vi "VS-Compute Heart Rate.vi"(0 "ECG":dbl[](array[numeric]), 7 "Sampling Rate (Hz)":dbl=10000.0, 11 "error in (no error)":errorcluster) -> (6 "Heart Rate (bpm)":dbl format="%.1f", 10 "XY Graph":cluster{"Array":dbl[], "Filtered X":dbl[]}[](graph), 15 "error out":errorcluster)   [LabVIEW 2020]
uses:
  <vilib>/Analysis/3filter.llb/Filter Passband Type.ctl
  epl-vi-lib/Utility VIs/Math VIs/LinSpace (x0-dx-npts).vi
  <vilib>/Analysis/baseanly.llb/Mean (DBL).vi
  <vilib>/Analysis/3filter.llb/Butterworth Filter (DBL).vi
  <vilib>/Analysis/NI_AALPro.lvlib
  <vilib>/Analysis/NI_AALBase.lvlib
  <vilib>/Analysis/NI_AAL_SigProc.lvlib
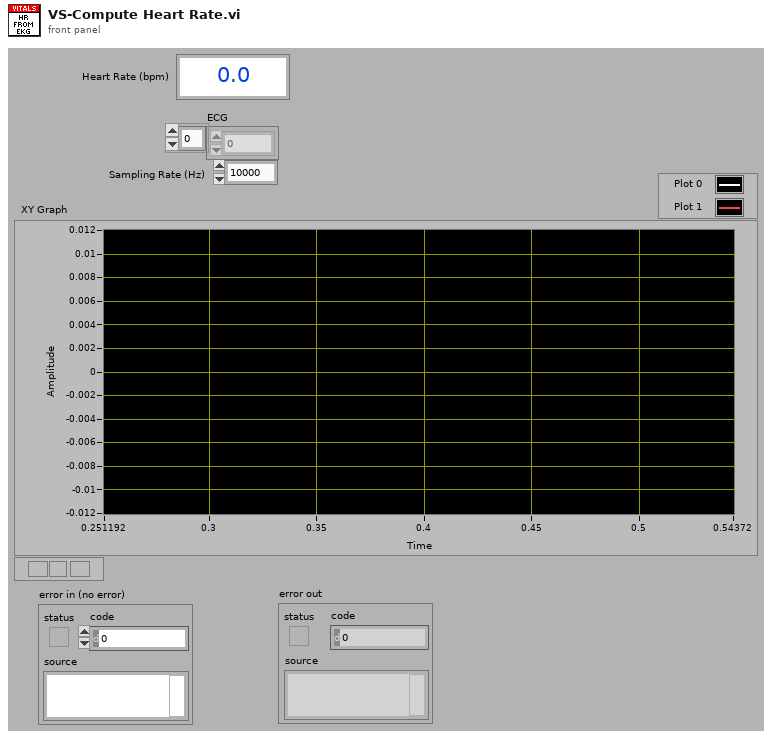
[diagram p1: front panel]
types:
  T1 = typedef "NI_AALBase.lvlib/Filter Passband Type.ctl" = enum32{"Lowpass", "Highpass", "Bandpass", "Bandstop"}
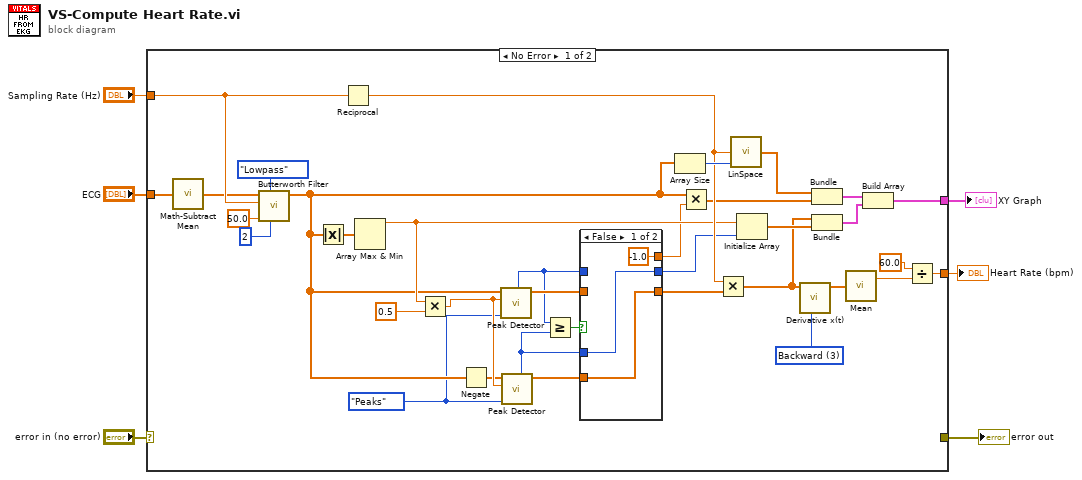
[diagram p0: block diagram]
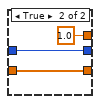
[diagram p2: hidden frame]
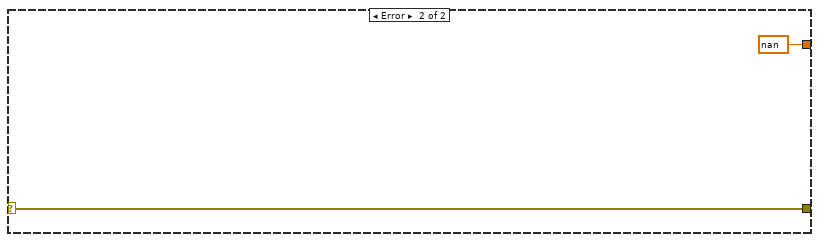
[diagram p3: hidden frame]
diagram:
  n1 = case shown="No Error" "error in (no error)" {
    selector: "error in (no error)" -> [_ w49]
    tunnel: [w41 nan] -> w6
    tunnel: "ECG" -> [w39 _]
    tunnel: "Sampling Rate (Hz)" -> [w37 _]
    tunnel: [_ w49] -> w2
    tunnel: [w10 _] -> w1
    frame No Error {
      w23 = u16 3 items=["2nd Order Central", "4th Order Central", "Forward", "Backward"] ("method")
      w7 = enum32{"Peaks", "Valleys"}."Peaks" ("peaks/valleys")
      n2 = call "Math-Subtract Mean.vi"("Y"=w39) -> ("Y - mean(Y)"=w29:dbl[])  [unwired: 4 in]
      n3 = call-poly <vilib>:"Butterworth Filter.vi"("order"=2, "filter type"=Filter_Passband_Type."Lowpass", "low cutoff freq: fl"=50.0, "sampling freq: fs"=w37, "X"=w29) -> ("Filtered X"=w19:dbl[])  [unwired: 3 in, 1 out]
      n4 = Absolute Value(x=w19) -> (abs(x)=w34:dbl[])
      n5 = Reciprocal(x=w37) -> (1/x=w28:dbl)
      n6 = Array Max & Min(array=w34) -> (max value=w27:dbl)  [unwired: 3 out]
      n7 = Multiply(x=w27, y=0.5) -> (x*y=w20:dbl)
      n8 = Negate(x=w19) -> (-x=w18:dbl[])
      n9 = call <vilib>:"Peak Detector.vi"("peaks/valleys"=w7, "threshold"=w20, "X"=w19) -> ("Locations"=w17:dbl[], "# found"=w14:i32)  [unwired: 4 in, 3 out]
      n10 = call <vilib>:"Peak Detector.vi"("peaks/valleys"=w7, "threshold"=w20, "X"=w18) -> ("Locations"=w16:dbl[], "# found"=w13:i32)  [unwired: 4 in, 3 out]
      n11 = Greater Or Equal?(x=w14, y=w13) -> (x >= y?=w15:bool)
      n12 = case shown="False" w15 {
        tunnel: w17 -> [_ w47]
        tunnel: w16 -> [w44 _]
        tunnel: w14 -> [_ w46]
        tunnel: w13 -> [w43 _]
        tunnel: [w44 w47] -> w12
        tunnel: [w43 w46] -> w11
        tunnel: [-1.0 1.0] -> w8
        frame False {
        }
        frame True {
        }
      }
      n13 = Array Size(array=w19) -> (size(s)=w32:i32)
      n14 = Multiply(x=w19, y=w8) -> (x*y=w9:dbl[])
      n15 = Multiply(x=w28, y=w12) -> (x*y=w22:dbl[])
      n16 = call-poly "LinSpace.vi"("npts"=w32, "dx"=w28) -> ("Array"=w31:dbl[])  [unwired: 2 in, 1 out]
      n17 = Initialize Array(w27, w11) -> (w25:dbl[])
      n18 = call <vilib>:"Derivative x(t).vi"("method"=w23, "X"=w22) -> ("dX/dt"=w24:dbl[])  [unwired: 8 in, 1 out]
      n19 = Bundle("Array"=w31, w9) -> (w30:cluster{"Array":dbl[], dbl[]})  [unwired: 1 in]
      n20 = Bundle(w22, w25) -> (w26:cluster{dbl[], dbl[]})  [unwired: 1 in]
      n21 = call-poly <vilib>:"Mean.vi"("X"=w24) -> ("mean"=w21:dbl)  [unwired: 1 out]
      n22 = Build Array(w30, w26) -> (w10:cluster{"Array":dbl[], dbl[]}[])
      n23 = Divide(x=60.0, y=w21) -> (x/y=w41:dbl)
    }
    frame Error {
    }
  }
  "Heart Rate (bpm)" <- w6
  "error out" <- w2
  "XY Graph" <- w1
